vi "Deactivate MastersHW.vi"(8 "error in (no error)":errorcluster, 11 "BME_DG_System in":refnum<class "BME_DG_System.lvclass">) -> (0 "error out":errorcluster, 2 "Deactivated?":bool, 3 "BME_DG_System out":refnum<class "BME_DG_System.lvclass">)   [LabVIEW 2009, in "POLARIS BME DG.lvlib" / "BME_DG_System.lvclass"]
uses:
  BME_DG_System.lvclass
  BME_DG_Base/BME_DG_Base.lvclass
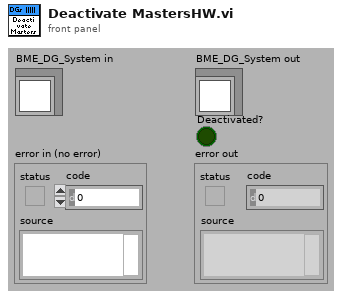
[diagram p1: front panel]
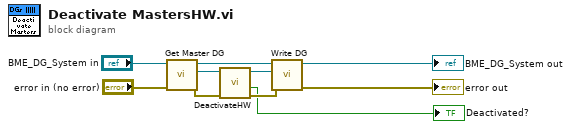
[diagram p0: block diagram]
diagram:
  n1 = call "Get Master DG.vi"("error in (no error)"="error in (no error)", "BME_DG_System in"="BME_DG_System in") -> ("error out"=w7:errorcluster, "BME_DG_Base.lvclass"=w8:refnum<class "BME_DG_Base.lvclass">, "BME_DG_System out"=w6:refnum<class "BME_DG_System.lvclass">)  [unwired: 7 in]
  n2 = call-dynamic "DeactivateHW.vi"("error in (no error)"=w7, "BME_DG_Base in"=w8) -> ("error out"=w3:errorcluster, "Deactivated?"=→"Deactivated?":bool, "BME_DG_Base out"=w4:refnum<class "BME_DG_Base.lvclass">)  [unwired: 6 in, 1 out]
  n3 = call "Write DG.vi"("error in (no error)"=w3, "BME_DG_Base"=w4, "BME_DG_System in"=w6) -> ("error out"=→"error out":errorcluster, "BME_DG_System out"=→"BME_DG_System out":refnum<class "BME_DG_System.lvclass">)  [unwired: 7 in]
